vi "esp301 set backlash.vi"(7 "Seperator in":string, 8 "error in (no error)":errorcluster, 9 "Args":string[](array[string]), 10 "String":string, 11 "ESP302 in":refnum<class "ESP302.lvclass">) -> (0 "error out":errorcluster, 2 "new commands":string, 3 "ESP302 out":refnum<class "ESP302.lvclass">)   [LabVIEW 2020, in "ESP302.lvclass"]
uses:
  ESP302.lvclass
  ESP302.lvclass/ESP302.ctl
  shared/CompressAndUpdate(Poly)/CompressAndUpdate(Numeric).vi
  ESP301/ESP301.lvclass
  C:/GEECS/Developers Version/source/Device Drivers/ESP301/ESP301.lvclass
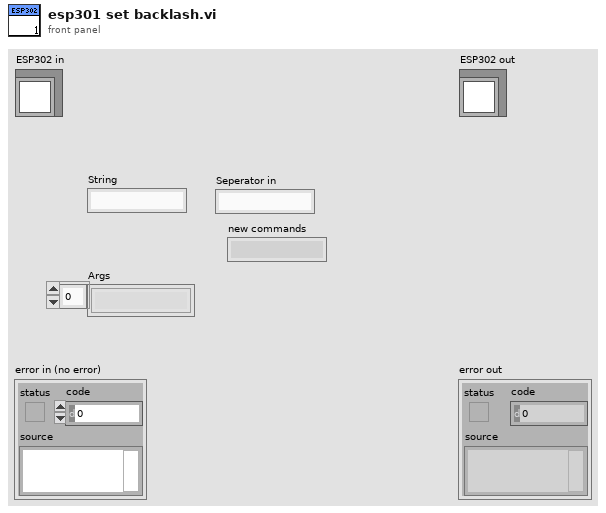
[diagram p1: front panel]
types:
  T1 = cluster{"Axis 1":cluster{"Value":dbl, "Min":dbl, "Max":dbl, "StepSize":dbl, "Tolerance":dbl, "ValueActual":dbl}, "Axis 2":cluster{"Value":dbl, "Min":dbl, "Max":dbl, "StepSize":dbl, "Tolerance":dbl, "ValueActual":dbl}, "Axis 3":cluster{"Value":dbl, "Min":dbl, "Max":dbl, "StepSize":dbl, "Tolerance":dbl, "ValueActual":dbl}}
  T2 = typedef "ESP301.lvclass/SettingsTypdef.ctl" = cluster{"devport":string, "Position":cluster{"Axis 1":cluster{"Value":dbl, "Min":dbl, "Max":dbl, "StepSize":dbl, "Tolerance":dbl, "ValueActual":dbl}, "Axis 2":cluster{"Value":dbl, "Min":dbl, "Max":dbl, "StepSize":dbl, "Tolerance":dbl, "ValueActual":dbl}, "Axis 3":cluster{"Value":dbl, "Min":dbl, "Max":dbl, "StepSize":dbl, "Tolerance":dbl, "ValueActual":dbl}}, "Power":cluster{"Axis 1":T3, "Axis 2":T3, "Axis 3":T3}, "Status":cluster{"Axis 1":T4, "Axis 2":T4, "Axis 3":T4}, "Backlash":cluster{"Axis 1":cluster{"Value":dbl, "Min":dbl, "Max":dbl, "StepSize":dbl, "Tolerance":dbl, "ValueActual":dbl}, "Axis 2":cluster{"Value":dbl, "Min":dbl, "Max":dbl, "StepSize":dbl, "Tolerance":dbl, "ValueActual":dbl}, "Axis 3":cluster{"Value":dbl, "Min":dbl, "Max":dbl, "StepSize":dbl, "Tolerance":dbl, "ValueActual":dbl}}, "Home":cluster{"Axis 1":cluster{"Value":dbl, "Min":dbl, "Max":dbl, "StepSize":dbl, "Tolerance":dbl, "ValueActual":dbl}, "Axis 2":cluster{"Value":dbl, "Min":dbl, "Max":dbl, "StepSize":dbl, "Tolerance":dbl, "ValueActual":dbl}, "Axis 3":cluster{"Value":dbl, "Min":dbl, "Max":dbl, "StepSize":dbl, "Tolerance":dbl, "ValueActual":dbl}}, "MoveToHardLimit":cluster{"Axis 1":T5, "Axis 2":T5, "Axis 3":T5}, "relativeMove":cluster{"Axis 1neg":T3, "Axis 2neg":T3, "Axis 3neg":T3, "Axis 1pos":T3, "Axis 2pos":T3, "Axis 3pos":T3}, "stepsize":cluster{"Value":dbl, "Min":dbl, "Max":dbl, "StepSize":dbl, "Tolerance":dbl, "ValueActual":dbl}, "automotoroff":T3, "ResetBeforeMove":T3, "Enable":cluster{"Axis 1":T3, "Axis 2":T3, "Axis 3":T3}}
  T3 = typedef "OnOffTypeDef.ctl" = enum16{"off", "on"}
  T4 = typedef "status_TypDef.ctl" = enum16{"Not referenced", "Homing", "Moving", "Ready"}
  T5 = typedef "Hardware limit.ctl" = enum16{"pos", "neg"}
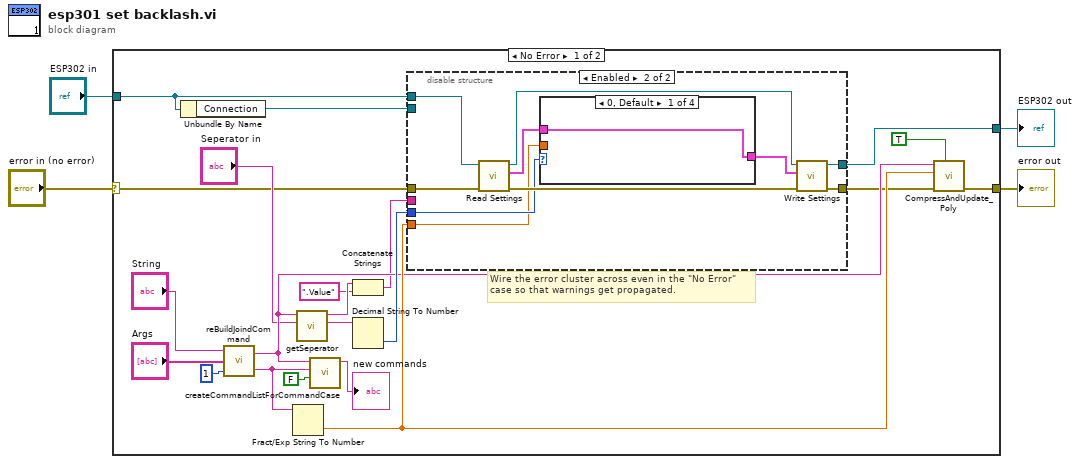
[diagram p0: block diagram]
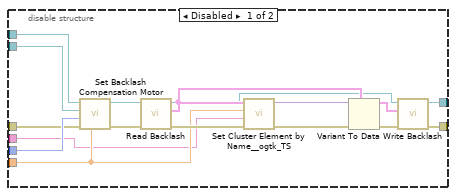
[diagram p2: hidden frame]
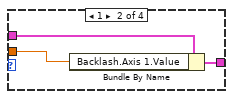
[diagram p3: hidden frame]
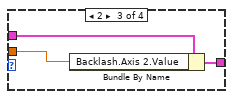
[diagram p4: hidden frame]
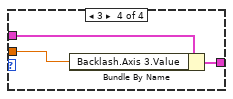
[diagram p5: hidden frame]
diagram:
  n1 = case shown="No Error" "error in (no error)" {
    selector: "error in (no error)" -> [w7 w64]
    tunnel: [w6 w64] -> w3
    tunnel: [w5 w63] -> w1
    tunnel: "ESP302 in" -> [w8 w63]
    frame No Error {
      # "Wire the error cluster across even in the \"No Error\"\ncase so that warnings get propagated."
      n2 = Unbundle By Name(w8) -> ("Connection"=w23:refnum<visa-resource-name>)
      n3 = call "reBuildJoindCommand.vi"("number of group elements (0)"=1, "Args"="Args", "Command 2"="String") -> ("Arg"=w21:string, "Command"=w22:string)
      n4 = Fract/Exp String To Number(string=w21) -> (number=w25:dbl)  [unwired: 3 in, 1 out]
      n5 = call "getSeperator.vi"("Channel Seperator (\"\")"="Seperator in", "Command"=w22) -> ("Channel"=w17:string, "Seperator (e.g. \"Channel1\")"=w19:string)  [unwired: 8 in]
      n6 = call "createCommandListForCommandCase.vi"("immediate Check (only once)"=FALSE, "setvalue"=w21, "command"=w22) -> ("new commands"=→"new commands":string)  [unwired: 8 in]
      n7 = Concatenate Strings(w19, ".Value" ("string")) -> (w20:string)
      n8 = Decimal String To Number(string=w17) -> (number=w24:i32)  [unwired: 2 in, 1 out]
      n9 = disable-structure shown="Enabled" {
        disable-tunnel: [w41 w47] -> w5
        disable-tunnel: w8 -> [w36 w52]
        disable-tunnel: w25 -> [w35 w43]
        disable-tunnel: w24 -> [w34 w44]
        disable-tunnel: w23 -> [w33 _]
        disable-tunnel: w7 -> [w32 w51]
        disable-tunnel: w20 -> [w29 _]
        disable-tunnel: [w27 w49] -> w9
        frame Disabled {
          n10 = call-dynamic "Set Backlash Compensation Motor.vi"("Backlash Compensation Value (0 units)"=w35, "error in (no error)"=w32, "Axis (1)"=w34, "VISA resource name"=w33, "ESP301 in"=w36) -> ("error out"=w39:errorcluster, "ESP301 out"=w37:refnum<class "ESP302.lvclass">)  [unwired: 4 in, 1 out]
          n11 = call "Read Backlash.vi"("error in (no error)"=w39, "ESP301 in"=w37) -> ("error out"=w40:errorcluster, "Backlash"=w38:T1, "ESP301 out"=w26:refnum<class "ESP302.lvclass">)  [unwired: 7 in]
          n12 = call "Set Cluster Element by Name__ogtk_TS.vi"("error in (no error)"=w40, "Element Name (\"\": New Element Data Name)"=w29, "New Element Value"=w35, "Cluster"=w38) -> ("error out"=w30:errorcluster, "VCluster out"=w31:variant)  [unwired: 5 in, 1 out]
          n13 = Variant To Data(error in=w30, type=w38, Variant=w31) -> (data=w42:T1, error out=w28:errorcluster)
          n14 = call "Write Backlash.vi"("error in (no error)"=w28, "Backlash"=w42, "ESP301 in"=w26) -> ("error out"=w27:errorcluster, "ESP301 out"=w41:refnum<class "ESP302.lvclass">)  [unwired: 7 in]
        }
        frame Enabled {
          n15 = call-dynamic "Read Settings.vi"("error in (no error)"=w51, "ESP301 in"=w52) -> ("error out"=w50:errorcluster, "Settings"=w46:T2, "ESP301 out"=w48:refnum<class "ESP302.lvclass">)  [unwired: 7 in]
          n16 = case shown="0, Default" w44 {
            tunnel: w46 -> [w53 w56 w59 w62]
            tunnel: [w53 w55 w58 w61] -> w45
            tunnel: w43 -> [_ w54 w57 w60]
            frame 0, Default {
            }
            frame 1 {
              n17 = Bundle By Name(cluster=w56, "Backlash.Axis 1.Value"=w54) -> (w55:T2)
            }
            frame 2 {
              n18 = Bundle By Name(cluster=w59, "Backlash.Axis 2.Value"=w57) -> (w58:T2)
            }
            frame 3 {
              n19 = Bundle By Name(cluster=w62, "Backlash.Axis 3.Value"=w60) -> (w61:T2)
            }
          }
          n20 = call-dynamic "Write Settings.vi"("error in (no error)"=w50, "Settings"=w45, "ESP301 in"=w48) -> ("error out"=w49:errorcluster, "ESP301 out"=w47:refnum<class "ESP302.lvclass">)  [unwired: 7 in]
        }
      }
      n21 = call-poly "CompressAndUpdate_Poly.vi"("force CVT update (false)"=TRUE ("force CVT update"), "error in"=w9, "Numeric"=w25, "command or variable name"=w22) -> ("error out"=w6:errorcluster)  [unwired: 7 in]
    }
    frame Error {
    }
  }
  "error out" <- w3
  "ESP302 out" <- w1
